vi "Dashboard Main.vi"() -> ()   [LabVIEW 2013]
uses:
  subStates.ctl
  <vilib>/event_ctls.llb/eventvkey.ctl
  Dashboard Datatype.ctl
  <vilib>/Rock Robotics/WPI/DriverStation/WPI_DriverStationDigitalData.ctl
  custom dash data.ctl
  vision data.ctl
  <vilib>/Rock Robotics/WPI/Joystick/WPI_JoystickButtonState.ctl
  <vilib>/Utility/config.llb/Write Key (String).vi
  <vilib>/Utility/config.llb/Write Key (I32).vi
  <vilib>/Utility/config.llb/NI_LVConfig.lvlib
panel:
  out "Image Message":string="Timeout in Camera Communications"
  in  "Dashboard Tab":T1(tab)
  out "vision calcs":bool
  out "arm saftey":bool
  out "arm encoder limit":bool
  out "pass?":bool
  out "hold":bool
  out "shoot?":bool
  out "Shifter":bool
  out "Vision State":bool
  out "Belts":dbl(knob) scale=-1.0..1.0
  in  "Camera Settings":T2={"Frame Rate"=30, "Compression"=30, "Size"=1} {"Frame Rate" scale=1.0..30.0; "Size" items=["640x480", "320x240", "160x120"]}
  out "Mode":T3(ring)=enum."Auto Disabled"
  out "Camera IP":string
  in  "DB Camera Config":bool
  out "fps":dbl format="%#.1g"
  out "Mbps":dbl format="%#.1g"
  out "Mbps 2":bool
  out "Distance From Target":dbl
  out "JS2 Z":dbl(slide) scale=-1.0..1.0 scale format="%#_2e"
  out "Joystick 2":cluster{"X":dbl, "Y":dbl}[](graph)
  out "JS Buttons 2":T4
  out "JS3 Z":dbl(slide) scale=-1.0..1.0 scale format="%#_2e"
  out "Joystick 3":cluster{"X":dbl, "Y":dbl}[](graph)
  out "JS Buttons 3":T4
  out "JS1 Z":dbl(slide) scale=-1.0..1.0 scale format="%#_2e"
  out "Joystick 1":cluster{"X":dbl, "Y":dbl}[](graph)
  out "JS Buttons 1":T4
  out "MotorChart L":T5(graph)
  out "MotorSliders L":T6 {"MotorSlide4 2" scale=0.0..14.0 scale format="%#_2e"; "MotorSlide2" scale=-1.0..1.0 scale format="%#_2e"; "MotorSlide1" scale=-1.0..1.0 scale format="%#_2e"}
  out "MotorChart R":cluster{"Numeric":dbl, "Numeric":dbl}(graph)
  out "MotorSliders R":cluster{"MotorSlide2":dbl, "MotorSlide1":dbl} {"MotorSlide1" scale=-1.0..1.0 scale format="%#_2e"; "MotorSlide2" scale=-1.0..1.0 scale format="%#_2e"}
  out "Drive":T7
  out "Shooter":T7
  out "Belts":T7
  out "Pickup Arm":T7
  out "Latch":T7
  out "Pickup/Passing \nArm":cluster{"Distance ":dbl, "Rate":dbl}
  out "Drive":cluster{"Right Motor":dbl, "Left Motor":dbl}
  out "Robot IP\nAddress":string
  out "Solenoid Output":bool[](array[boolean])
  out "PWM":cluster{u8, u8}[](array[slide])=[{0, 157}, {0, 157}, {0, 157}, {0, 157}, {0, 157}, {0, 157}, {0, 157}, {0, 157}, {0, 157}, {0, 169}] scale=1.0..255.0
  out "GPIO Output Enable":bool[](array[boolean])
  out "GPIO State":bool[](array[boolean])
  out "Relay":cluster{"Forward":bool[], "Reverse":bool[]}
  out "8 -- Battery":sgl(graph)
  out "Analog Input":sgl[](array[slide]) scale=0.0..5.0
  out "cRIO CPU Usage":dbl(knob) scale=0.0..100.0
  out "Code Iterations Per Second":cluster{dbl, dbl}(knob) scale=0.0..60.0
  out "Vision mSPI":u32
  out "Main mSPI":u32
  in  "Listbox":i32(listbox)
  out "Tree":string(tree)
  out "Camera Image":T8(plugin-control)
  in  "Enable":bool
  # "ft"
  # "Joysticks"
  # "Encoders"
  # "Drive and Battery"
  # "States"
  # "Left"
  # "Front"
  # "Right"
  # "Battery"
  # "Communications"
  # "Solenoid #1"
  # "1"
  # "8"
  # "Digital #1"
  # "1"
  # "10"
  # "1"
  # "14"
  # "1"
  # "8"
  # "Analog #1"
  # "1"
  # "7"
  # "Main IPS"
  # "Vision IPS"
  # "Grey - Vision\nBlack - Main"
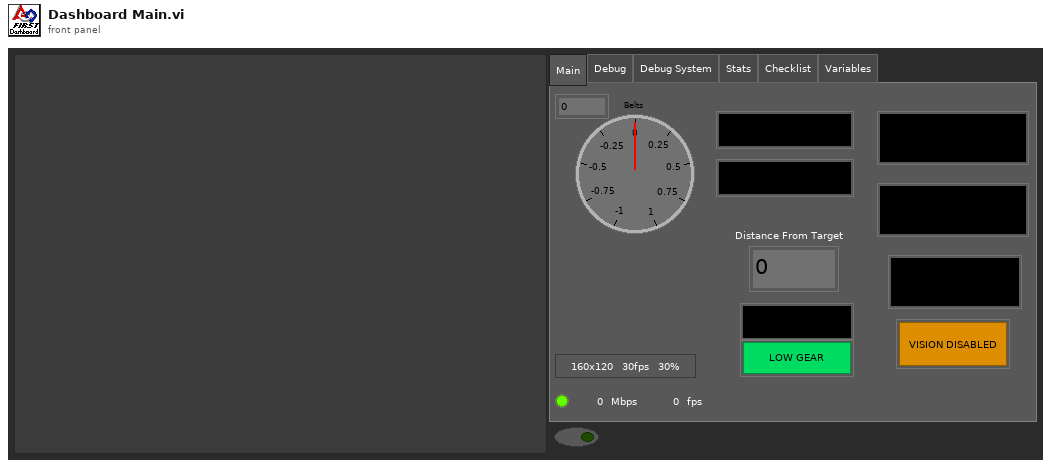
[diagram p1: front panel]
types:
  T1 = enum32{"Main", "Debug", "Debug System", "Stats", "Checklist", "Variables"}
  T2 = cluster{"Frame Rate":i32, "Compression":i32, "Size":u16}
  T3 = enum8{"Tele-Op Disabled", "Tele-Op Enabled", "Auto Disabled", "Auto Enabled", "Test Disabled", "Test Enabled", ""}
  T4 = cluster{bool, bool, bool, bool, bool, bool, bool, bool, bool, bool, bool, bool}
  T5 = cluster{"Numeric":dbl, "Numeric":dbl, "Battery":sgl}
  T6 = cluster{"MotorSlide1":dbl, "MotorSlide2":dbl, "MotorSlide4 2":dbl}
  T7 = typedef "subStates.ctl" = enum16{"null", "wait", "driver control", "auto", "manual override", "hold position", "rotate", "pickup", "pass", "load", "goto shoot", "shoot", "end"}
  T8 = typedef "IMAQ Image.ctl" = refnum<image>
  T9 = typedef "Image Type" = u32
  T10 = typedef "custom dash data.ctl" = cluster{"Motors":cluster{"Pickup Motor":dbl, "Pickup Belt":dbl, "Pickup Distance ":dbl, "Pickup Rate":dbl, "Right Motor":dbl, "Left Motor":dbl}, "substates":cluster{"Latch":T7, "Pickup Arm":T7, "Belts":T7, "Shooter":T7, "Drive":T7}, "Safeties":cluster{"Arm Safety":bool, "Arm Limit":bool}, "Performance":cluster{"CPU Usage":dbl, "Vision mSPI":u32, "Main mSPI":u32}, "Data":T11, "Joysticks":cluster{"J1 Axes":cluster{"axis 1 (x)":dbl, "axis 2 (y)":dbl, "axis 3 (throttle)":dbl, "axis 4":dbl, "axis 5":dbl, "axis 6":dbl}, "J1 Buttons":T12, "J2 Axes":cluster{"axis 1 (x)":dbl, "axis 2 (y)":dbl, "axis 3 (throttle)":dbl, "axis 4":dbl, "axis 5":dbl, "axis 6":dbl}, "J2 Buttons":T12, "J3 Axes":cluster{"axis 1 (x)":dbl, "axis 2 (y)":dbl, "axis 3 (throttle)":dbl, "axis 4":dbl, "axis 5":dbl, "axis 6":dbl}, "J3 Buttons":T12}, "SubSystem Manager":cluster{"Ball State Read":enum16{"no ball", "holding", "loaded"}, "Picked Up":bool, "Loaded":bool, "Shooter Cocked":bool, "Arm Ready":bool}, "Vision Enabled?":bool}
  T11 = typedef "vision data.ctl" = cluster{"x":dbl, "y":dbl, "area":dbl, "width":dbl, "height":dbl, "Hot Goal Present?":bool, "distance":dbl}
  T12 = typedef "WPI_JoystickButtonState.ctl" = cluster{"Button 1":bool, "Button 2":bool, "Button 3":bool, "Button 4":bool, "Button 5":bool, "Button 6":bool, "Button 7":bool, "Button 8":bool, "Button 9":bool, "Button 10":bool, "Button 11":bool, "Button 12":bool}
  T13 = typedef "Dashboard Datatype.ctl" = cluster{cluster{"AnalogModule[0]":cluster{"Channel[0]":sgl, "Channel[1]":sgl, "Channel[2]":sgl, "Channel[3]":sgl, "Channel[4]":sgl, "Channel[5]":sgl, "Channel[6]":sgl, "Channel[7]":sgl}, "AnalogModule[1]":cluster{"Channel[0]":sgl, "Channel[1]":sgl, "Channel[2]":sgl, "Channel[3]":sgl, "Channel[4]":sgl, "Channel[5]":sgl, "Channel[6]":sgl, "Channel[7]":sgl}}, cluster{"DigitalModule[0]":T14, "DigitalModule[1]":T14}, "Solenoid":u8}
  T14 = typedef "WPI_DriverStationDigitalData.ctl" = cluster{"Relay Fwd":u8, "Relay Rev":u8, "GPIO":u16, "GPIO_OE":u16, "PWM":cluster{"PWM[0]":u8, "PWM[1]":u8, "PWM[2]":u8, "PWM[3]":u8, "PWM[4]":u8, "PWM[5]":u8, "PWM[6]":u8, "PWM[7]":u8, "PWM[8]":u8, "PWM[9]":u8}}
  T15 = cluster{"Digital Inputs":bool[], "Digital Outputs":bool[]}
  T16 = cluster{"Competition mode":bool, "Robot Link":bool, "Autonomous":bool, "Enabled":bool, "E-Stop":bool, "Simulated":bool, "TestMode":bool, "Docked Window":bool}
  T17 = cluster{"J1 Axes":cluster{"axis 1 (x)":dbl, "axis 2 (y)":dbl, "axis 3 (throttle)":dbl, "axis 4":dbl, "axis 5":dbl, "axis 6":dbl}, "J1 Buttons":T12, "J2 Axes":cluster{"axis 1 (x)":dbl, "axis 2 (y)":dbl, "axis 3 (throttle)":dbl, "axis 4":dbl, "axis 5":dbl, "axis 6":dbl}, "J2 Buttons":T12, "J3 Axes":cluster{"axis 1 (x)":dbl, "axis 2 (y)":dbl, "axis 3 (throttle)":dbl, "axis 4":dbl, "axis 5":dbl, "axis 6":dbl}, "J3 Buttons":T12}
  T18 = cluster{"Pickup Motor":dbl, "Pickup Belt":dbl, "Pickup Distance ":dbl, "Pickup Rate":dbl, "Right Motor":dbl, "Left Motor":dbl}
  T19 = cluster{"Latch":T7, "Pickup Arm":T7, "Belts":T7, "Shooter":T7, "Drive":T7}
  T20 = cluster{"CPU Usage":dbl, "Vision mSPI":u32, "Main mSPI":u32}
  T21 = cluster{"AnalogModule[0]":cluster{"Channel[0]":sgl, "Channel[1]":sgl, "Channel[2]":sgl, "Channel[3]":sgl, "Channel[4]":sgl, "Channel[5]":sgl, "Channel[6]":sgl, "Channel[7]":sgl}, "AnalogModule[1]":cluster{"Channel[0]":sgl, "Channel[1]":sgl, "Channel[2]":sgl, "Channel[3]":sgl, "Channel[4]":sgl, "Channel[5]":sgl, "Channel[6]":sgl, "Channel[7]":sgl}}
  T22 = cluster{"DigitalModule[0]":T14, "DigitalModule[1]":T14}
  T23 = cluster{"Left Motor":dbl, "Left Motor":dbl, "Battery":sgl}
  T24 = cluster{"Pickup Distance ":dbl, "Pickup Rate":dbl}
  T25 = cluster{"Channel[0]":sgl, "Channel[1]":sgl, "Channel[2]":sgl, "Channel[3]":sgl, "Channel[4]":sgl, "Channel[5]":sgl, "Channel[6]":sgl, "Channel[7]":sgl}[]
  T26 = cluster{"Channel[0]":sgl, "Channel[1]":sgl, "Channel[2]":sgl, "Channel[3]":sgl, "Channel[4]":sgl, "Channel[5]":sgl, "Channel[6]":sgl, "Channel[7]":sgl}
  T27 = cluster{"axis 1 (x)":dbl, "axis 2 (y)":dbl, "axis 3 (throttle)":dbl, "axis 4":dbl, "axis 5":dbl, "axis 6":dbl}
  T28 = typedef "NI_LVConfig.lvlib/Config Data RefNum.ctl" = refnum<k1>
  T29 = typedef "eventvkey.ctl" = enum16{"ASCII", "Enter", "Return", "Shift", "Ctrl", "Alt", "Cmd", "Opt", "Caps", "NumLock", "Clear", "Break", "Up", "Down", "Left", "Right", "Insert", "Delete", "Home", "End", "PageUp", "PageDown", "Escape", "Help", "Pause", "ScrollLock", "F1", "F2", "F3", "F4", "F5", "F6", "F7", "F8", "F9", "F10", "F11", "F12", "F13", "F14", "F15", "F16", "F17", "F18", "F19", "F20", "F21", "F22", "F23", "F24", "Play", "VolumeUp", "VolumeDown", "Mute", "Two Byte Char"}
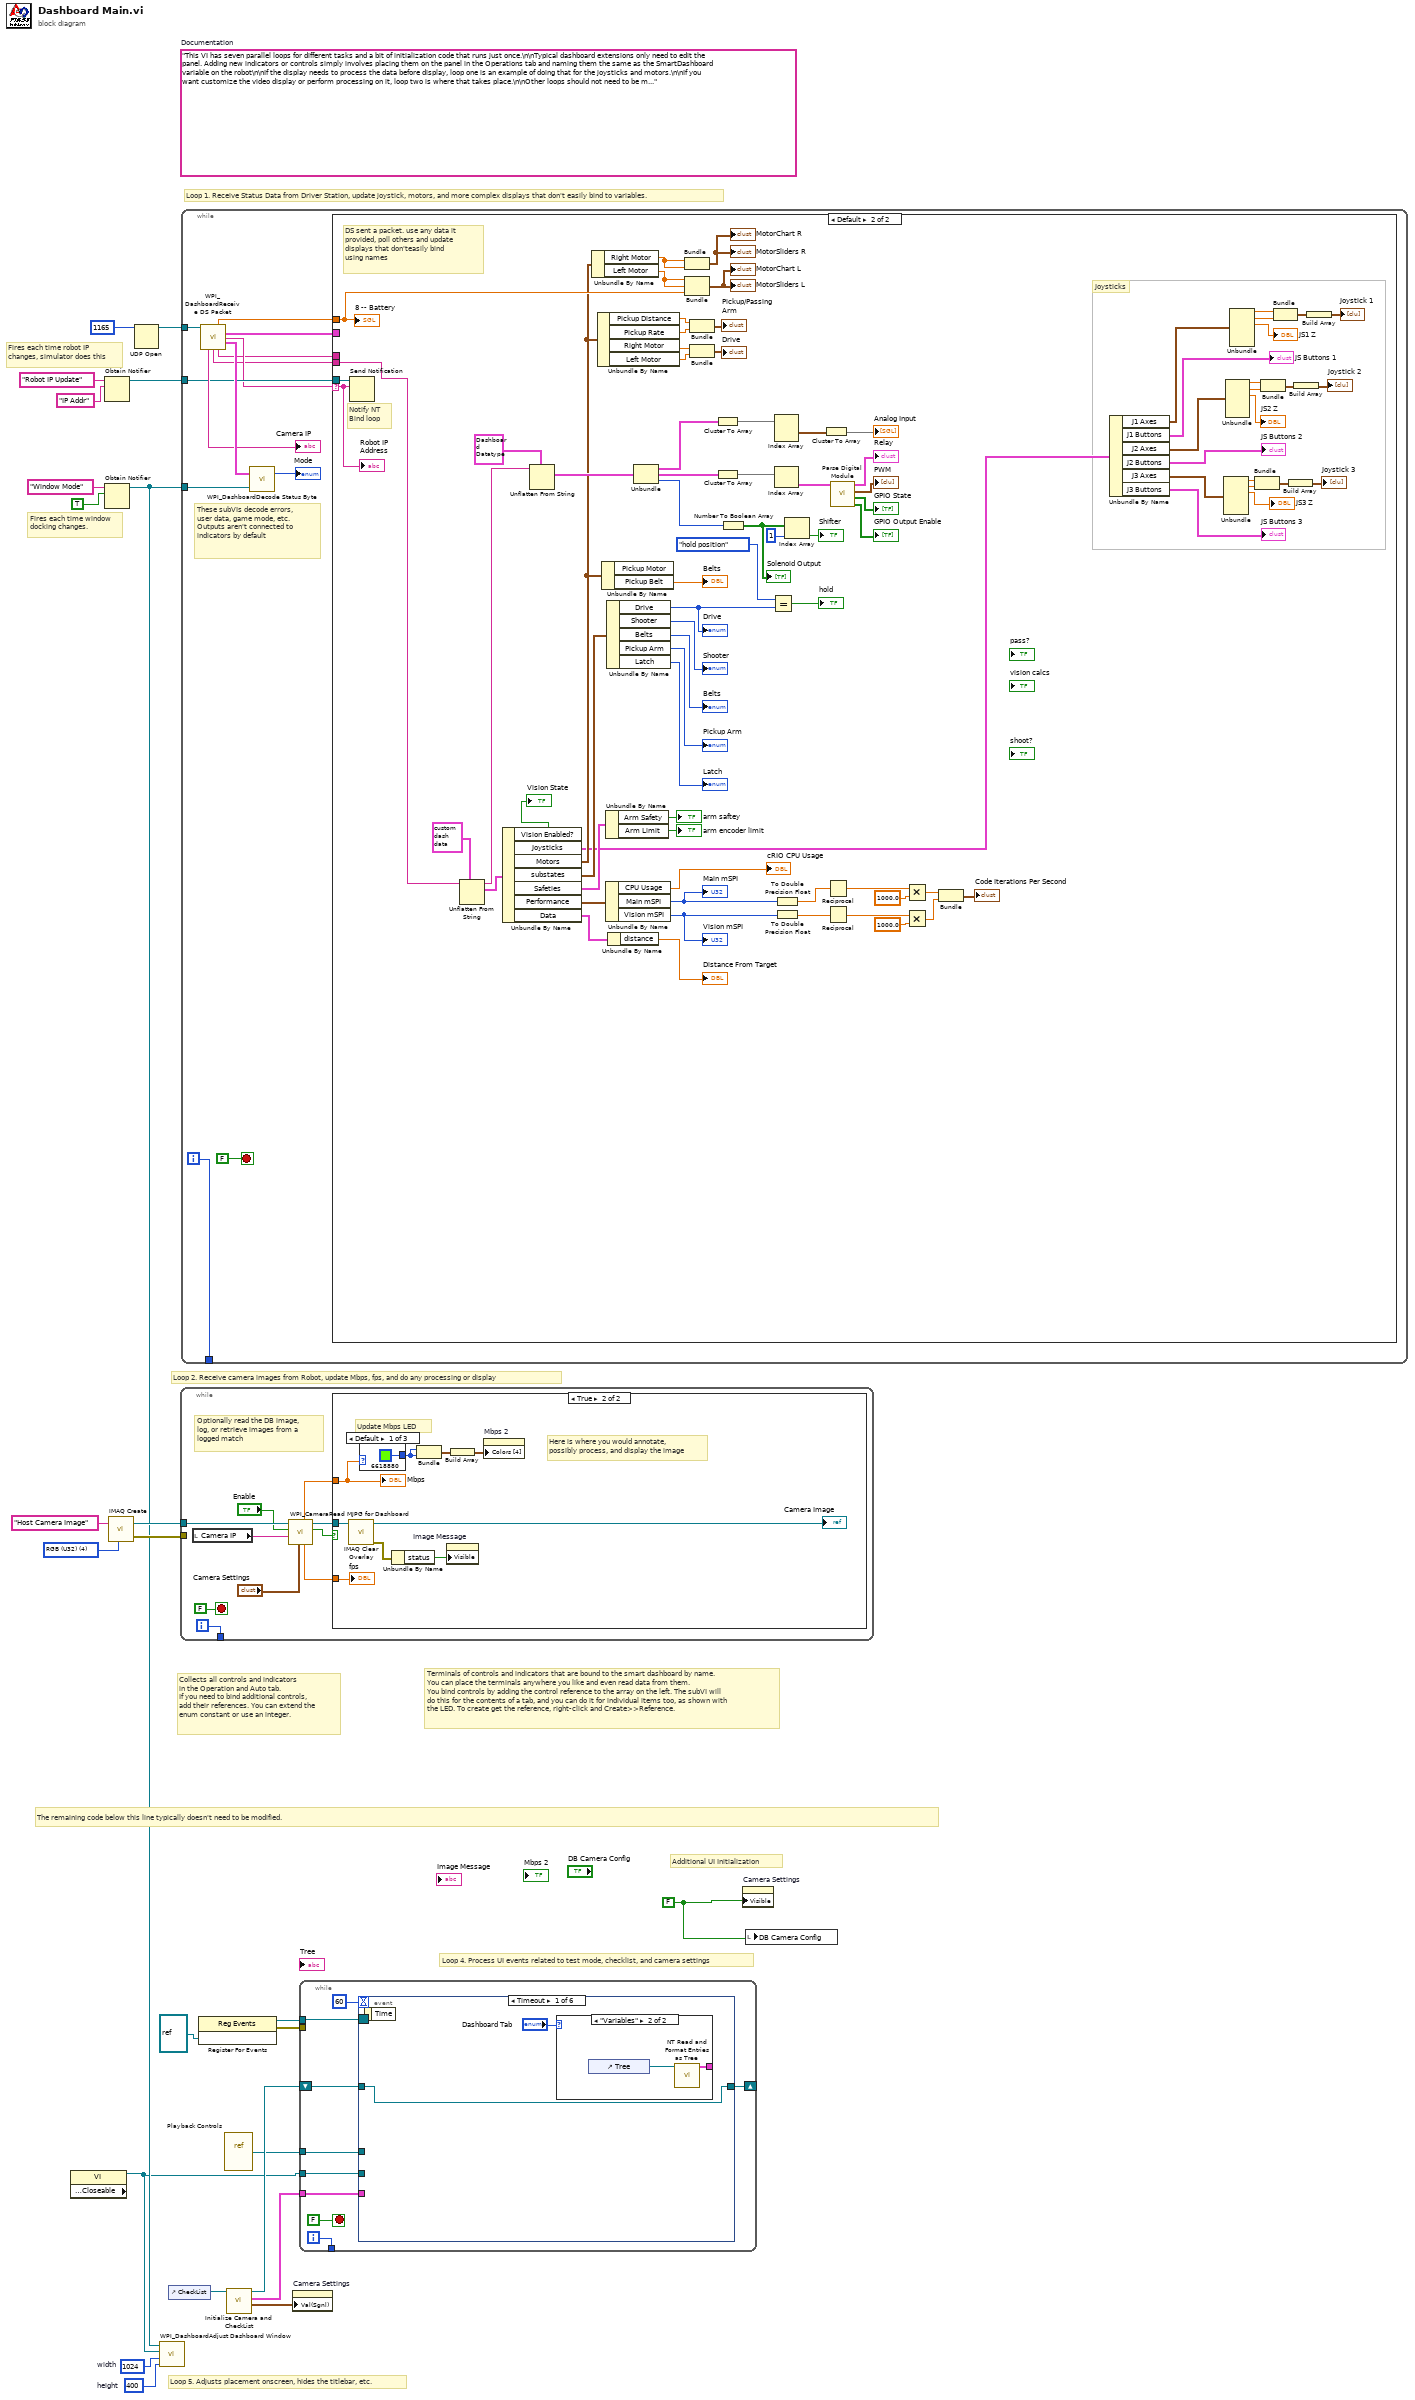
[diagram p0: block diagram]
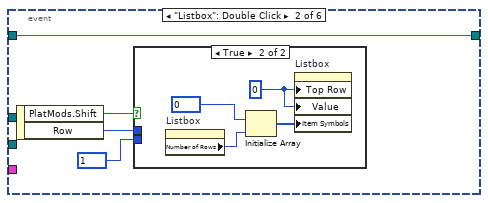
[diagram p3: hidden frame]
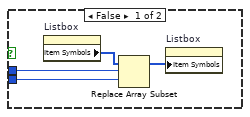
[diagram p4: hidden frame]
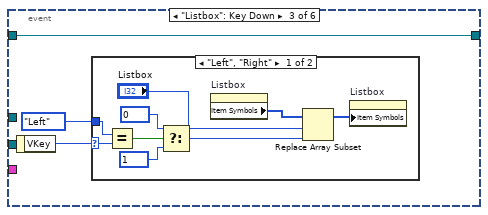
[diagram p5: hidden frame]
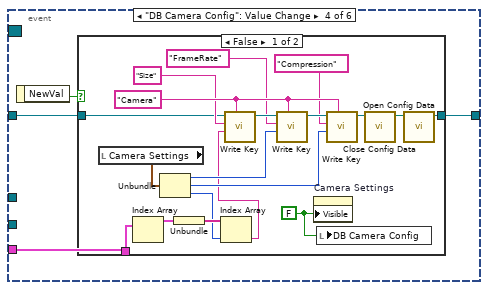
[diagram p7: hidden frame]
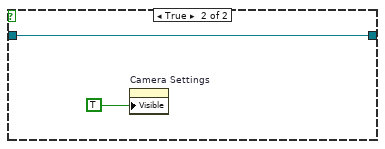
[diagram p8: hidden frame]
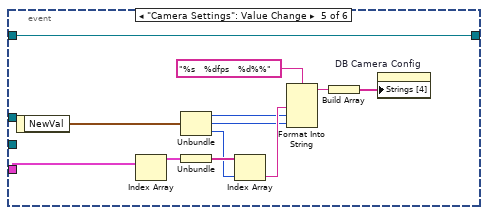
[diagram p9: hidden frame]
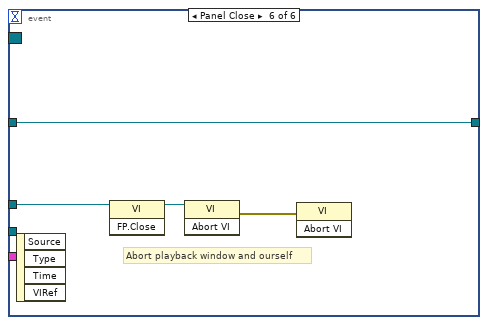
[diagram p10: hidden frame]
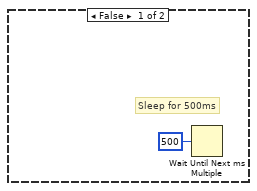
[diagram p11: hidden frame]
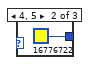
[diagram p12: hidden frame]
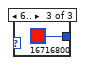
[diagram p13: hidden frame]
diagram:
  w3 = 400  # height
  w4 = 1024  # width
  w13 = FALSE ("Visible")
  (unwired) "This VI has seven parallel loops for different tasks and a bit of initialization code that runs just once.\n\nTypical dashboard extensions only need to edit the panel. Adding new indicators or controls simply involves placing them on the panel in the Operations tab and naming them the same as the SmartDashboard variable on the robot\n\nIf the display needs to process the data before display, loop one is an example of doing that for the joysticks and motors.\n\nIf you want customize the video display or perform processing on it, loop two is where that takes place.\n\nOther loops should not need to be modified. They are pretty standard, and document the task they perform."  # Documentation
  w22 = T9 4 items=["Grayscale (U8)", "Grayscale (I16)", "Grayscale (SGL)", "Complex (CSG)", "RGB (U32)", "HSL (U32)", "RGB (U64)"] ("Image Type")
  # "Loop 4. Process UI events related to test mode, checklist, and camera settings"
  # "Loop 5. Adjusts placement onscreen, hides the titlebar, etc."
  # "Additional UI Initialization"
  # "Fires each time robot IP\nchanges, simulator does this"
  # "Fires each time window\ndocking changes."
  # "Collects all controls and indicators\nin the Operation and Auto tab.\nIf you need to bind additional controls,\nadd their references. You can extend the\nenum constant or use an integer."
  # "The remaining code below this line typically doesn't need to be modified."
  # "Terminals of controls and indicators that are bound to the smart dashboard by name.\nYou can place the terminals anywhere you like and even read data from them.\nYou bind controls by adding the control reference to the array on the left. The subVI will\ndo this for the contents of a tab, and you can do it for individual items too, as shown with\nthe LED. To create get the reference, right-click and Create>>Reference."
  # "Loop 1. Receive Status Data from Driver Station, update joystick, motors, and more complex displays that don't easily bind to variables."
  # "Loop 2. Receive camera images from Robot, update Mbps, fps, and do any processing or display"
  n1 = property class="VI" props=["Front Panel.Closeable"]() -> (reference out=w1:refnum<vi>)  [unwired: 2 in, 2 out]
  n2 = Obtain Notifier(name (unnamed)="Robot IP Update", notification data type="IP Addr" ("name (unnamed)")) -> (notifier out=w16:refnum<notifier>)  [unwired: 2 in, 2 out]
  n3 = Obtain Notifier(name (unnamed)="Window Mode", notification data type=TRUE) -> (notifier out=w12:refnum<notifier>)  [unwired: 2 in, 2 out]
  n4 = call "IMAQ Create"("Image Name"="Host Camera Image", "Image Type"=w22) -> ("New Image"=w20:T8, "error out"=w19:errorcluster)  [unwired: 2 in, 1 out]
  n5 = UDP Open(11:u16 1165 ("port")) -> (port=w23:refnum<k16>)  [unwired: 2 in, 4 out]
  n6 = call <vilib>:"WPI_DashboardAdjust Dashboard Window.vi"("height"=w3, "width"=w4, "reference in"=w1, "Notifier in"=w12) -> ()  [unwired: 8 in]
  n7 = control-ref of="CheckList"() -> (w2:refnum<vi>)
  n8 = while {
    tunnel: w20 -> [w32]
    tunnel: w19 -> [_]
    tunnel: [w33] -> _
    i -> [w33]
    stop <- FALSE stop-if-true
    # "Optionally read the DB image,\nlog, or retrieve images from a\nlogged match"
    n9 = local read "Camera IP"() -> (w25:string)
    n10 = call <vilib>:"WPI_CameraRead MJPG for Dashboard.vi"("Camera Settings"="Camera Settings", "Camera IP"=w25, "Enable"="Enable", "Refnum in"=w32) -> ("Active"=w29:bool, "Refnum out"=w31:T8, "FPS"=w28:dbl, "Bandwidth (Mbps)"=w27:dbl)  [unwired: 4 in]
    n11 = case shown="True" w29 {
      tunnel: w31 -> [_ w39]
      tunnel: w27 -> [_ w38]
      tunnel: w28 -> [_ w36]
      frame False {
        # "Sleep for 500ms"
        n12 = Wait Until Next ms Multiple(millisecond multiple=u32 500) -> ()  [unwired: 1 out]
      }
      frame True {
        # "Here is where you would annotate,\npossibly process, and display the image"
        # "Update Mbps LED"
        n13 = call "IMAQ Clear Overlay"("Image"=w39) -> ("error out"=w43:errorcluster, "Image Out"=→"Camera Image":T8)  [unwired: 2 in, 7 out]
        n14 = case shown="Default" w38 {
          tunnel: [u32 6618880 ("Color Box") u32 16776722 ("Color Box") u32 16716800 ("Color Box")] -> w40
          frame Default {
          }
          frame 4, 5 {
          }
          frame 6.. {
          }
        }
        n15 = Unbundle By Name(w43) -> ("status"=w44:bool)
        n16 = Bundle("Color Box"=w40, "Color Box"=w40) -> (w42:cluster{"Color Box":u32, "Color Box":u32})  [unwired: 1 out]
        n17 = property on="Image Message" class="Str"("Visible"=w44) -> ()  [unwired: 2 in, 2 out]
        n18 = Build Array(w42) -> (w41:cluster{"Color Box":u32, "Color Box":u32}[])
        n19 = property on="Mbps 2" class="Bool (strict)"("Colors [4]"=w41) -> ()  [unwired: 2 in, 2 out]
        "Mbps" <- w38
        "fps" <- w36
      }
    }
  }
  n20 = while {
    tunnel: w23 -> [w58]
    tunnel: w16 -> [w53]
    tunnel: w12 -> [w57]
    tunnel: [w54] -> _
    i -> [w54]
    stop <- FALSE stop-if-true
    # "These subVIs decode errors, user data, game mode, etc.\nOutputs aren't connected to indicators by default"
    n21 = call <vilib>:"WPI_DashboardReceive DS Packet.vi"("Recv Socket"=w58) -> ("Battery"=w48:sgl, "Driver Station"=w49:T15, "Robot IP Address"=w52:string, "Status"=w59:T16, "Camera IP Address"=→"Camera IP":string, "Low Priority User Data"=w51:string, "High Priority User Data"=w50:string)  [unwired: 1 in, 7 out]
    n22 = call <vilib>:"WPI_DashboardDecode Status Byte.vi"("Window Mode Notifier"=w57, "Status"=w59) -> ("Mode"=→"Mode":T3)  [unwired: 1 out]
    n23 = case shown="Default" w52 {
      selector: w52 -> [_ w103]
      tunnel: w53 -> [_ w144]
      tunnel: w51 -> [_ w130]
      tunnel: w50 -> [_ _]
      tunnel: w49 -> [_ _]
      tunnel: w48 -> [_ w109]
      frame "0.0.0.0" {
        # "DS not sending packets, or no robot exists yet.\nDon't poll the variables"
      }
      frame Default {
        # "Joysticks"
        # "Notify NT\nBind loop"
        # "DS sent a packet. use any data it\nprovided, poll others and update\ndisplays that don'teasily bind\nusing names"
        n24 = Send Notification(notification=w103, notifier=w144) -> ()  [unwired: 1 in, 2 out]
        n25 = Unflatten From String(type=T10 {"Motors"={"Pickup Motor"=0.0, "Pickup Belt"=0.0, "Pickup Distance "=0.0, "Pickup Rate"=0.0, "Right Motor"=0.0, "Left Motor"=0.0}, "substates"={"Latch"=enum."null", "Pickup Arm"=enum."null", "Belts"=enum."null", "Shooter"=enum."null", "Drive"=enum."null"}, "Safeties"={"Arm Safety"=FALSE, "Arm Limit"=FALSE}, "Performance"={"CPU Usage"=0.0, "Vision mSPI"=0, "Main mSPI"=0}, "Data"={"x"=0.0, "y"=0.0, "area"=0.0, "width"=0.0, "height"=0.0, "Hot Goal Present?"=FALSE, "distance"=0.0}, "Joysticks"={"J1 Axes"={"axis 1 (x)"=0.0, "axis 2 (y)"=0.0, "axis 3 (throttle)"=0.0, "axis 4"=0.0, "axis 5"=0.0, "axis 6"=0.0}, "J1 Buttons"={"Button 1"=FALSE, "Button 2"=FALSE, "Button 3"=FALSE, "Button 4"=FALSE, "Button 5"=FALSE, "Button 6"=FALSE, "Button 7"=FALSE, "Button 8"=FALSE, "Button 9"=FALSE, "Button 10"=FALSE, "Button 11"=FALSE, "Button 12"=FALSE}, "J2 Axes"={"axis 1 (x)"=0.0, "axis 2 (y)"=0.0, "axis 3 (throttle)"=0.0, "axis 4"=0.0, "axis 5"=0.0, "axis 6"=0.0}, "J2 Buttons"={"Button 1"=FALSE, "Button 2"=FALSE, "Button 3"=FALSE, "Button 4"=FALSE, "Button 5"=FALSE, "Button 6"=FALSE, "Button 7"=FALSE, "Button 8"=FALSE, "Button 9"=FALSE, "Button 10"=FALSE, "Button 11"=FALSE, "Button 12"=FALSE}, "J3 Axes"={"axis 1 (x)"=0.0, "axis 2 (y)"=0.0, "axis 3 (throttle)"=0.0, "axis 4"=0.0, "axis 5"=0.0, "axis 6"=0.0}, "J3 Buttons"={"Button 1"=FALSE, "Button 2"=FALSE, "Button 3"=FALSE, "Button 4"=FALSE, "Button 5"=FALSE, "Button 6"=FALSE, "Button 7"=FALSE, "Button 8"=FALSE, "Button 9"=FALSE, "Button 10"=FALSE, "Button 11"=FALSE, "Button 12"=FALSE}}, "SubSystem Manager"={"Ball State Read"=enum."no ball", "Picked Up"=FALSE, "Loaded"=FALSE, "Shooter Cocked"=FALSE, "Arm Ready"=FALSE}, "Vision Enabled?"=FALSE} ("Custom Dash Data"), binary string=w130) -> (rest of the binary string=w128:string, value=w136:T10)  [unwired: 3 in, 1 out]
        n26 = Unbundle By Name(w136) -> ("Vision Enabled?"=→"Vision State":bool, "Joysticks"=w78:T17, "Motors"=w79:T18, "substates"=w114:T19, "Safeties"=w117:cluster{"Arm Safety":bool, "Arm Limit":bool}, "Performance"=w98:T20, "Data"=w135:T11)
        n27 = Unflatten From String(type=T13 {{"AnalogModule[0]"={"Channel[0]"=0.0, "Channel[1]"=0.0, "Channel[2]"=0.0, "Channel[3]"=0.0, "Channel[4]"=0.0, "Channel[5]"=0.0, "Channel[6]"=0.0, "Channel[7]"=0.0}, "AnalogModule[1]"={"Channel[0]"=0.0, "Channel[1]"=0.0, "Channel[2]"=0.0, "Channel[3]"=0.0, "Channel[4]"=0.0, "Channel[5]"=0.0, "Channel[6]"=0.0, "Channel[7]"=0.0}}, {"DigitalModule[0]"={"Relay Fwd"=0, "Relay Rev"=0, "GPIO"=0, "GPIO_OE"=0, "PWM"={"PWM[0]"=0, "PWM[1]"=0, "PWM[2]"=0, "PWM[3]"=0, "PWM[4]"=0, "PWM[5]"=0, "PWM[6]"=0, "PWM[7]"=0, "PWM[8]"=0, "PWM[9]"=0}}, "DigitalModule[1]"={"Relay Fwd"=0, "Relay Rev"=0, "GPIO"=0, "GPIO_OE"=0, "PWM"={"PWM[0]"=0, "PWM[1]"=0, "PWM[2]"=0, "PWM[3]"=0, "PWM[4]"=0, "PWM[5]"=0, "PWM[6]"=0, "PWM[7]"=0, "PWM[8]"=0, "PWM[9]"=0}}}, "Solenoid"=0} ("Dashboard Data"), binary string=w128) -> (value=w127:T13)  [unwired: 3 in, 2 out]
        n28 = Unbundle By Name(w79) -> ("Right Motor"=w132:dbl, "Left Motor"=w133:dbl)
        n29 = Unbundle By Name(w79) -> ("Pickup Distance"=w84:dbl, "Pickup Rate"=w85:dbl, "Right Motor"=w82:dbl, "Left Motor"=w81:dbl)
        n30 = Unbundle By Name(w79) -> ("Pickup Belt"=→"Belts":dbl)  [unwired: 1 out]
        n31 = Unbundle By Name(w117) -> ("Arm Safety"=→"arm saftey":bool, "Arm Limit"=→"arm encoder limit":bool)
        n32 = Unbundle By Name(w98) -> ("CPU Usage"=→"cRIO CPU Usage":dbl, "Main mSPI"=w94:u32, "Vision mSPI"=w90:u32)
        "Vision mSPI" <- w90
        "Main mSPI" <- w94
        n33 = Unbundle By Name(w114) -> ("Drive"=w113:T7, "Shooter"=→"Shooter":T7, "Belts"=→"Belts":T7, "Pickup Arm"=→"Pickup Arm":T7, "Latch"=→"Latch":T7)
        "Drive" <- w113
        n34 = Unbundle By Name(w135) -> ("distance"=→"Distance From Target":dbl)
        n35 = Unbundle(w127) -> (w121:T21, w123:T22, "Solenoid"=w120:u8)
        n36 = Bundle("Right Motor"=w132, "Right Motor"=w132) -> (→"MotorChart R" →"MotorSliders R":cluster{"Right Motor":dbl, "Right Motor":dbl})  [unwired: 1 in]
        n37 = Bundle("Left Motor"=w133, "Left Motor"=w133, "Battery"=w109) -> (→"MotorChart L" →"MotorSliders L":T23)  [unwired: 1 in]
        n38 = Bundle("Pickup Distance"=w84, "Pickup Rate"=w85) -> (→"Pickup/Passing \nArm":T24)  [unwired: 1 in]
        n39 = Bundle("Right Motor"=w82, "Left Motor"=w81) -> (→"Drive":cluster{"Right Motor":dbl, "Left Motor":dbl})  [unwired: 1 in]
        n40 = Cluster To Array(cluster=w121) -> (array=w124:T25)
        n41 = Cluster To Array(cluster=w123) -> (array=w125:T14[])
        n42 = Number To Boolean Array(number=w120) -> (Boolean array=w108:bool[])
        "Solenoid Output" <- w108
        n43 = Equal?(x=subStates."hold position" ("Drive"), y=w113) -> (x = y?=→"hold":bool)
        n44 = Index Array(array=w124) -> (element #1=w126:T26)  [unwired: 2 in, 1 out]
        n45 = Index Array(array=w125) -> (element=w122:T14)  [unwired: 1 in]
        n46 = To Double Precision Float(number=w94) -> (double precision float=w97:dbl)
        n47 = To Double Precision Float(number=w90) -> (double precision float=w91:dbl)
        n48 = Index Array(array=w108, index=1) -> (element=→"Shifter":bool)
        n49 = Cluster To Array(cluster=w126) -> (array=→"Analog Input":sgl[])
        n50 = Reciprocal(x=w97) -> (1/x=w96:dbl)
        n51 = Reciprocal(x=w91) -> (1/x=w92:dbl)
        n52 = call "Parse Digital Module.vi"("DigitalModule"=w122) -> ("GPIO Output Enable"=→"GPIO Output Enable":bool[], "GPIO State"=→"GPIO State":bool[], "PWM"=→"PWM":cluster{u8, u8}[], "Relay"=→"Relay":cluster{"Forward":bool[], "Reverse":bool[]})  [unwired: 7 in]
        n53 = Multiply(x=w96, y=1000.0) -> (x*y=w89:dbl)
        n54 = Multiply(x=w92, y=1000.0) -> (x*y=w88:dbl)
        n55 = Bundle(w89, w88) -> (→"Code Iterations Per Second":cluster{dbl, dbl})  [unwired: 1 in]
        n56 = Unbundle By Name(w78) -> ("J1 Axes"=w77:T27, "J1 Buttons"=→"JS Buttons 1":T12, "J2 Axes"=w69:T27, "J2 Buttons"=→"JS Buttons 2":T12, "J3 Axes"=w64:T27, "J3 Buttons"=→"JS Buttons 3":T12)
        n57 = Unbundle(w64) -> ("axis 1 (x)"=w67:dbl, "axis 2 (y)"=w66:dbl, "axis 3 (throttle)"=→"JS3 Z":dbl)  [unwired: 3 out]
        n58 = Unbundle(w69) -> ("axis 1 (x)"=w70:dbl, "axis 2 (y)"=w71:dbl, "axis 3 (throttle)"=→"JS2 Z":dbl)  [unwired: 3 out]
        n59 = Unbundle(w77) -> ("axis 1 (x)"=w76:dbl, "axis 2 (y)"=w74:dbl, "axis 3 (throttle)"=→"JS1 Z":dbl)  [unwired: 3 out]
        n60 = Bundle("axis 1 (x)"=w67, "axis 2 (y)"=w66) -> (w138:cluster{"axis 1 (x)":dbl, "axis 2 (y)":dbl})  [unwired: 1 in]
        n61 = Bundle("axis 1 (x)"=w70, "axis 2 (y)"=w71) -> (w140:cluster{"axis 1 (x)":dbl, "axis 2 (y)":dbl})  [unwired: 1 in]
        n62 = Bundle("axis 1 (x)"=w76, "axis 2 (y)"=w74) -> (w145:cluster{"axis 1 (x)":dbl, "axis 2 (y)":dbl})  [unwired: 1 in]
        n63 = Build Array(w138) -> (→"Joystick 3":cluster{"axis 1 (x)":dbl, "axis 2 (y)":dbl}[])
        n64 = Build Array(w140) -> (→"Joystick 2":cluster{"axis 1 (x)":dbl, "axis 2 (y)":dbl}[])
        n65 = Build Array(w145) -> (→"Joystick 1":cluster{"axis 1 (x)":dbl, "axis 2 (y)":dbl}[])
        "8 -- Battery" <- w109
        "Robot IP\nAddress" <- w103
      }
    }
  }
  n66 = register-events(refnum<vi> refnum) -> (reference out=w7:refnum<event-registration>, error out=w6:errorcluster)  [unwired: 2 in]
  n67 = vi-ref "Playback Controls.vi"() -> (w8:refnum<vi>)
  n68 = call "Initialize Camera and CheckList.vi"("ListBox in"=w2) -> ("Cluster"=w10:cluster{"value":i32, "value":i32, "index":i32}, "Array"=w11:cluster{string[]}[], "File Refnum"=w9:T28)  [unwired: 8 in]
  n69 = property on="Camera Settings" class="Clust (strict)"("Val(Sgnl)"=w10) -> ()  [unwired: 2 in, 2 out]
  n70 = while {
    tunnel: w11 -> [w152]
    shift-right: [w151] -> _
    shift-left: w9 -> [w150]
    tunnel: [w149] -> _
    tunnel: w8 -> [w148]
    tunnel: w7 -> [w147]
    tunnel: w6 -> [_]
    tunnel: w1 -> [w146]
    i -> [w149]
    stop <- FALSE stop-if-true
    n71 = event shown="[0] Timeout" {
      selector: w147 -> [_ _ _ _ _ _]
      dyn-events: _ -> [_ _ _ _ _ _]
      timeout: u32 60 ("milliseconds to wait") -> [_ _ _ _ _ _]
      tunnel: w152 -> [_ _ _ w185 w215 _]
      tunnel: [w155 w159 w171 w184 w208 w220] -> w151
      tunnel: w150 -> [w155 w159 w171 w183 w208 w220]
      tunnel: w148 -> [_ _ _ _ _ w223]
      tunnel: w146 -> [_ _ _ _ _ _]
      event Timeout {
        n72 = event-data() -> ()  [unwired: 1 in, 1 out]
        n73 = case shown="\"Variables\"" "Dashboard Tab" {
          tunnel: [_ w158] -> _
          frame "Debug", Default {
          }
          frame "Variables" {
            n74 = control-ref of="Tree"() -> (w157:refnum<vi>)
            n75 = call <vilib>:"NT Read and Format Entries as Tree.vi"("Tree Refnum"=w157) -> ("Formatted Strings"=w158:cluster{"Name":string, "Value":string}[])  [unwired: 9 in, 1 out]
          }
        }
      }
      event "Listbox": Double Click {
        n76 = event-data() -> ("PlatMods.Shift"=w160:bool, "Row"=w162:i32)  [unwired: 1 in]
        n77 = case shown="True" w160 {
          tunnel: w162 -> [w166 _]
          tunnel: 1 -> [w165 _]
          frame False {
            n78 = property on="Listbox" class="LstBox (strict)"() -> ("Item Symbols"=w164:i32[])  [unwired: 2 in, 2 out]
            n79 = Replace Array Subset(array=w164, new element=w165, index=w166) -> (w163:i32[])
            n80 = property on="Listbox" class="LstBox (strict)"("Item Symbols"=w163) -> ()  [unwired: 2 in, 2 out]
          }
          frame True {
            w167 = 0 ("Top Row")
            n81 = property on="Listbox" class="LstBox (strict)"() -> ("Number of Rows"=w169:u32)  [unwired: 2 in, 2 out]
            n82 = Initialize Array(0, w169) -> (w168:i32[])
            n83 = property on="Listbox" class="LstBox (strict)"("Top Row"=w167, "Value"=w167, "Item Symbols"=w168) -> ()  [unwired: 2 in, 2 out]
          }
        }
      }
      event "Listbox": Key Down {
        n84 = event-data() -> ("VKey"=w173:T29)  [unwired: 1 in]
        n85 = case shown="\"Left\", \"Right\"" w173 {
          selector: w173 -> [w178 _]
          tunnel: eventvkey."Left" ("VKey") -> [w176 _]
          frame "Left", "Right" {
            n86 = Equal?(x=w176, y=w178) -> (x = y?=w177:bool)
            n87 = Select(t=0, s=w177, f=1) -> (s? t:f=w179:i32)
            n88 = property on="Listbox" class="LstBox (strict)"() -> ("Item Symbols"=w182:i32[])  [unwired: 2 in, 2 out]
            n89 = Replace Array Subset(array=w182, new element=w179, index="Listbox") -> (w181:i32[])
            n90 = property on="Listbox" class="LstBox (strict)"("Item Symbols"=w181) -> ()  [unwired: 2 in, 2 out]
          }
          frame Default {
          }
        }
      }
      event "DB Camera Config": Value Change {
        n91 = event-data() -> ("NewVal"=w186:bool)  [unwired: 1 in]
        n92 = case shown="False" w186 {
          tunnel: w185 -> [w195 _]
          tunnel: [w188 w206] -> w184
          tunnel: w183 -> [w187 w206]
          frame False {
            w202 = "Camera"
            w205 = FALSE ("Visible")
            n93 = local read "Camera Settings"() -> (w194:T2)
            n94 = Index Array(array=w195) -> (element=w198:cluster{string[]})  [unwired: 1 in]
            n95 = Unbundle(w194) -> ("Frame Rate"=w193:i32, "Compression"=w192:i32, "Size"=w196:u16)
            n96 = Unbundle(w198) -> (w197:string[])
            n97 = Index Array(array=w197, index=w196) -> (element=w191:string)
            n98 = call-poly <vilib>:"Write Key.vi"("section"=w202, "value"=w191, "key"="Size", "refnum"=w187) -> ("refnum out"=w204:T28)  [unwired: 2 in, 5 out]
            n99 = call-poly <vilib>:"Write Key.vi"("section"=w202, "value"=w193, "key"="FrameRate", "refnum"=w204) -> ("refnum out"=w203:T28)  [unwired: 1 in, 6 out]
            n100 = property on="Camera Settings" class="Clust (strict)"("Visible"=w205) -> ()  [unwired: 2 in, 2 out]
            n101 = local write "DB Camera Config"(w205) -> ()
            n102 = call-poly <vilib>:"Write Key.vi"("section"=w202, "value"=w192, "key"="Compression", "refnum"=w203) -> ("refnum out"=w189:T28)  [unwired: 1 in, 6 out]
            n103 = call <vilib>:"Close Config Data.vi"("refnum"=w189) -> ("file path"=w190:path)  [unwired: 2 in, 8 out]
            n104 = call <vilib>:"Open Config Data.vi"("configuration file path"=w190) -> ("refnum"=w188:T28)  [unwired: 8 in, 2 out]
          }
          frame True {
            n105 = property on="Camera Settings" class="Clust (strict)"("Visible"=TRUE) -> ()  [unwired: 2 in, 2 out]
          }
        }
      }
      event "Camera Settings": Value Change {
        n106 = event-data() -> ("NewVal"=w219:T2)  [unwired: 1 in]
        n107 = Index Array(array=w215) -> (element=w214:cluster{string[]})  [unwired: 1 in]
        n108 = Unbundle(w219) -> ("Frame Rate"=w210:i32, "Compression"=w209:i32, "Size"=w212:u16)
        n109 = Unbundle(w214) -> (w213:string[])
        n110 = Index Array(array=w213, index=w212) -> (element=w211:string)
        n111 = Format Into String(format string="%s   %dfps   %d%%", w211, w210, w209) -> (resulting string=w216:string)  [unwired: 2 in, 1 out]
        n112 = Build Array(w216) -> (w217:string[])
        n113 = property on="DB Camera Config" class="Bool (strict)"("Strings [4]"=w217) -> ()  [unwired: 2 in, 2 out]
      }
      event Panel Close {
        # "Abort playback window and ourself"
        n114 = event-data() -> ()  [unwired: 1 in, 4 out]
        n115 = invoke class="VI" method="FP.Close"(reference=w223) -> (reference out=w222:refnum<vi>)  [unwired: 2 in, 2 out]
        n116 = invoke class="VI" method="Abort VI"(reference=w222) -> (error out=w221:errorcluster)  [unwired: 2 in, 2 out]
        n117 = invoke class="VI" method="Abort VI"(error in=w221) -> ()  [unwired: 2 in, 3 out]
      }
    }
  }
  n118 = property on="Camera Settings" class="Clust (strict)"("Visible"=w13) -> ()  [unwired: 2 in, 2 out]
  n119 = local write "DB Camera Config"(w13) -> ()
